vi "GetSecond.vi"(10 "String in":string) -> (2 "String out":string)   [LabVIEW 2019]
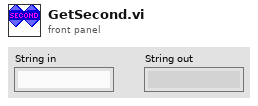
[diagram p1: front panel]
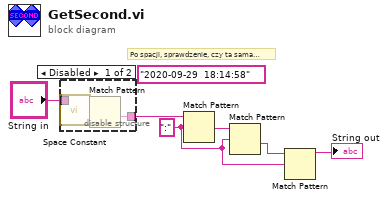
[diagram p0: block diagram]
diagram:
  (unwired) "2020-09-29  18:14:58"
  w2 = ":" ("regular expression")
  # "Po spacji, sprawdzenie, czy ta sama sekunda"
  n1 = disable-structure shown="Disabled" {
    disable-tunnel: "String in" -> [w9 w10]
    disable-tunnel: [w7 w10] -> w4
    frame Disabled {
      n2 = call <vilib>:"Space Constant.vi"() -> ("String"=w8:string)
      n3 = Match Pattern(string=w9, regular expression=w8) -> (after substring=w7:string)  [unwired: 1 in, 3 out]
    }
    frame Enabled {
    }
  }
  n4 = Match Pattern(string=w4, regular expression=w2) -> (after substring=w3:string)  [unwired: 1 in, 3 out]
  n5 = Match Pattern(string=w3, regular expression=w2) -> (after substring=w1:string)  [unwired: 1 in, 3 out]
  n6 = Match Pattern(string=w1, regular expression=w2) -> (before substring=→"String out":string)  [unwired: 1 in, 3 out]
